vi "Add Constant to 2D Array Column.vi"(9 "column":i32=1, 10 "2D Array":dbl[][](array[numeric]), 11 "Constant":dbl) -> (3 "Power Time Array out":dbl[][](array[numeric]))   [LabVIEW 2017]
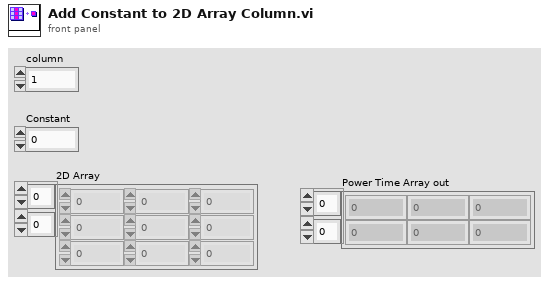
[diagram p1: front panel]
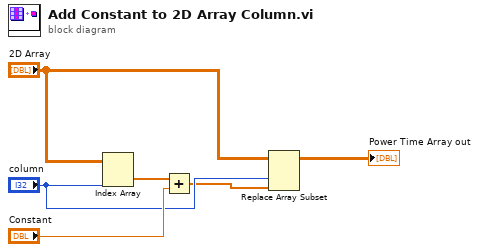
[diagram p0: block diagram]
diagram:
  n1 = Index Array(array="2D Array", index (col)="column") -> (element=w5:dbl[])  [unwired: 1 in]
  n2 = Add(x=w5, y="Constant") -> (x+y=w2:dbl[])
  n3 = Replace Array Subset(array="2D Array", new element=w2, index (col)="column") -> (→"Power Time Array out":dbl[][])  [unwired: 1 in]
